vi "Main.vi"() -> ()   [LabVIEW 2018, in "Settings.lvlib"]
doc: "This template is based off of the Queued Message Handler design pattern and the Queued Message Handler project template that ships with LabVIEW.\n\nThe main difference is that the queue is private to this module and communication between modules is performed via Broadcast and Request events.\n\nRequest events are wrapped in public API methods and are handled in the Event Handling Loop (EHL) of this VI. Any module can register for Broadcast events sent by this module. The EHL generates messages based on user interface actions.\n\nThe Message Handling Loop (MHL) processes messages generated by the EHL, or by other messages. The messages are string values, so new messages can be added easily to the Message Cases case structure in the MHL. Each message cluster can also provide an optional value for Message Data, which is a variant that can be converted to whatever message-specific data is required.\n_____\nBased on Delacor QMH Project Template 4.2.1.64."
uses:
  Settings.lvlib
  <vilib>/Delacor/Delacor QMH/Libraries/Module Admin_class/Delacor_lib_QMH_Module Admin.lvclass
  Private API/Data.lvclass
  <vilib>/Delacor/Delacor QMH/Libraries/Message Queue_class/Delacor_lib_QMH_Message Queue.lvclass/Delacor_lib_QMH_Message Queue.ctl
  Stop Argument--cluster.ctl
  <vilib>/Delacor/Delacor QMH/Libraries/Module Admin_class/Delacor_lib_QMH_Module Admin.lvclass/Delacor_lib_QMH_Module Admin.ctl
  Load Settings from File Argument--cluster.ctl
  Instant Load Settings from File Argument--cluster.ctl
  Instant Load Settings from File (Reply Payload)--cluster.ctl
  Common/Typedefs/CTL_Settings_cluster_2.ctl
  SubVi's/Controls/CTL_Histogram_parameters.ctl
  SubVi's/Controls/CTL_Filter_selector.ctl
  SubVi's/Controls/CTL_Acquisition_speed_selector.ctl
  Common/Typedefs/CTL_Segmented_plot_parameters_2.ctl
  Cage Diagram/Typedefs/CTL_Cage_type.ctl
  SubVi's/Controls/CTL_Cage_all_segmentation_params_set.ctl
  SubVi's/Controls/CTL_IO_params_cluster.ctl
  SubVi's/Controls/CTL_Conditions_Array.ctl
  SubVi's/Controls/CTL_Conditions_Cluster.ctl
  SubVi's/Controls/CTL_Condition_type.ctl
  SubVi's/Controls/CTL_Comparison_type.ctl
  SubVi's/Controls/CTL_Validity_check_criteria.ctl
  SubVi's/Controls/CTL_Response_info.ctl
  SubVi's/Controls/CTL_Condition_response_type.ctl
  SubVi's/Controls/CTL_Reponse_port_info.ctl
  SubVi's/Controls/CTL_Calibration_parameters.ctl
  SubVi's/Controls/CTL_Dispenser_calibration_info.ctl
  <vilib>/Utility/miscctls.llb/LVPointTypeDef.ctl
  Private API/Data.lvclass/Data.ctl
  <vilib>/Delacor/Delacor QMH/Libraries/Message Queue_class/Delacor_lib_QMH_Enqueue Message (Single).vi
  <vilib>/Delacor/Delacor QMH/Libraries/Module Admin_class/Delacor_lib_QMH_Get External Launch.vi
  Private API/Methods/Write Status.vi
  <vilib>/Utility/error.llb/Error Cluster From Error Code.vi
  <vilib>/ErrorRing/Error Ring.xnode
  <vilib>/Delacor/Delacor QMH/Libraries/Message Queue_class/Delacor_lib_QMH_Message Queue.lvclass
  Common_Resources.lvlib
  Cage Diagram/Cage Diagram.lvlib
panel:
  out "Settings path to load":path
  in  "Simulate MHL Error":bool
  in  "Simulate EHL Error":bool
  out "error out":errorcluster
  in  "Module Admin":refnum<class "Delacor_lib_QMH_Module Admin.lvclass">
  out "Status":string
  # "Settings Module"
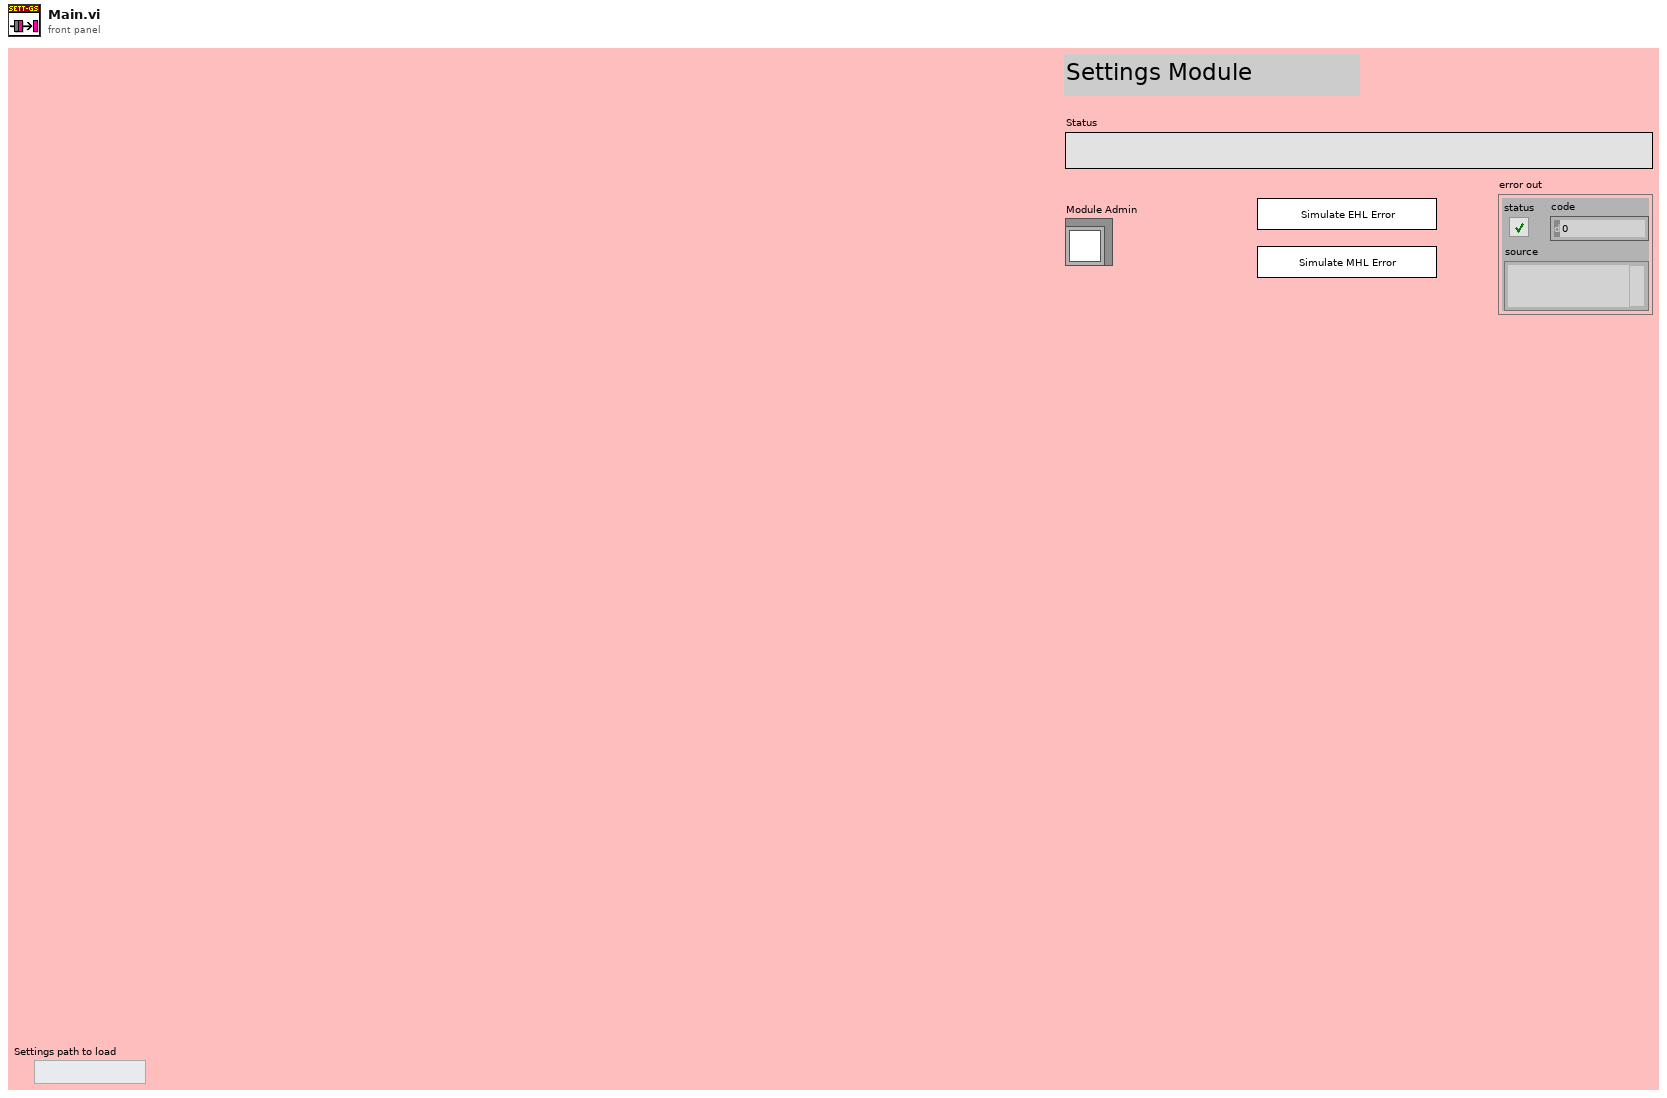
[diagram p1: front panel]
types:
  T1 = typedef "Settings.lvlib/Request Events--cluster.ctl" = cluster{"Stop Module":refnum<user-event>, "Show Panel":refnum<user-event>, "Hide Panel":refnum<user-event>, "Get Module Execution Status":refnum<user-event>, "Show Diagram":refnum<user-event>, "Load Settings from File":refnum<user-event>, "Instant Load Settings from File":refnum<user-event>}
  T2 = enum32{"invalid lock state", "Not Locked", "Locked (No Password)", "Password-protected"}
  T3 = typedef "Settings.lvlib/Stop Argument--cluster.ctl" = cluster{"Origin":string, "Exit via Stop Module Req?":bool, "Wait for Module to stop?":bool}
  T4 = typedef "Settings.lvlib/Load Settings from File Argument--cluster.ctl" = cluster{"Path: Default or Custom?":bool, "Settings File Path":path, "Researcher name":string}
  T5 = typedef "Settings.lvlib/Instant Load Settings from File Argument--cluster.ctl" = cluster{"Path: Default or Custom?":bool, "Settings File Path":path, "Researcher name":string, "Wait Notifier":refnum<notifier>, "wait for reply":bool}
  T6 = typedef "LVPointTypeDef.ctl" = cluster{"Horizontal":i16, "Vertical":i16}
  T7 = enum32{"Invalid", "Standard", "Closed", "Hidden", "Minimized", "Maximized"}
  T8 = typedef "Settings.lvlib/Instant Load Settings from File (Reply Payload)--cluster.ctl" = cluster{"Settings cluster":T9, "Instant Load Settings from File_error":errorcluster}
  T9 = typedef "Common_Resources.lvlib/CTL_Settings_cluster_2.ctl" = cluster{"Defaults":cluster{"Default User":dbl, "VISA Resource Name ":string, "Histogram parameters":T10}, "Recording and saving":cluster{"Researcher name":string, "Name prefix":string, "Data post-processing":T11, "Stop at":dbl, "\"Stop at\" enabled":bool, "Default save folder path":path, "Acquisition FPS":T12}, "Geometry":T13, "IO parameters":T16, "Conditions presets array":T17, "Calibration parameters":T25}
  T10 = typedef "Common_Resources.lvlib/CTL_Histogram_parameters.ctl" = cluster{"max":dbl, "min":dbl, "# bins":i32, "threshold":dbl, "thr. type":enum16{"higher accepted", "lower accepted"}}
  T11 = typedef "Common_Resources.lvlib/CTL_Filter_selector.ctl" = cluster{"Filter type":enum16{"None", "Savitzky-Golay"}, "Length":i32, "Order":i32}
  T12 = typedef "Common_Resources.lvlib/CTL_Acquisition_speed_selector.ctl" = enum16{"Max", "Optimal", "Eco"}
  T13 = typedef "Common_Resources.lvlib/CTL_Segmented_plot_parameters_2.ctl" = cluster{"Sensor board size":enum16{"", "Large"}, "Bridge swap":bool, "Twisted neck":bool, "Bridge H. offset":sgl, "Bridge V. offset":sgl, "Magnets orientation":sgl, "Cage type":T14, "Cage parameters":T15}
  T14 = typedef "Cage Diagram.lvlib/CTL_Cage_type.ctl" = u16
  T15 = typedef "Common_Resources.lvlib/CTL_Cage_all_segmentation_params_set.ctl" = cluster{"Round":variant, "Square":variant, "Donut-maze":variant, "T-maze":variant, "Sociability-maze":variant}
  T16 = typedef "Common_Resources.lvlib/CTL_IO_params_cluster.ctl" = cluster{"IO general config.":u16, "IO 1 configuration":u16, "IO 2 configuration":u16, "IO 3 configuration":u16, "IO 4 configuration":u16, "Activate ext. RS-232":u16, "IO inversion config.":u16, "Sync capability":u8}
  T17 = typedef "Common_Resources.lvlib/CTL_Conditions_Array.ctl" = T18[]
  T18 = typedef "Common_Resources.lvlib/CTL_Conditions_Cluster.ctl" = cluster{"Enabled":bool, "Name":string, "Specifier(s)":cluster{"Specifier enabled":bool, "Condition type":T19, "Comparison type":T20, "Value":dbl, "Validity criteria(s)":cluster{"V. check enabled":bool, "Criteria":T21, "Validity value":dbl}[]}[], "Response":T22, "Has been set":bool}
  T19 = typedef "Common_Resources.lvlib/CTL_Condition_type.ctl" = enum16{"Speed", "Zone", "Angle to wall"}
  T20 = typedef "Common_Resources.lvlib/CTL_Comparison_type.ctl" = enum16{"Less", "Less or Equal", "Equal", "Greater or Equal", "Greater", "Not Equal"}
  T21 = typedef "Common_Resources.lvlib/CTL_Validity_check_criteria.ctl" = enum16{"Running bout (seconds)", "Running bout (meters)"}
  T22 = typedef "Common_Resources.lvlib/CTL_Response_info.ctl" = cluster{"Response type":T23, "TTL port":T24, "TTL pulse length, ms":dbl}
  T23 = typedef "Common_Resources.lvlib/CTL_Condition_response_type.ctl" = enum16{"None", "Air puff", "Liquid reward", "TTL pulse", "TTL pulse (ubr)", "TTL signal"}
  T24 = typedef "Common_Resources.lvlib/CTL_Reponse_port_info.ctl" = enum16{"Port 1", "Port 2", "Port 3", "Port 4"}
  T25 = typedef "Common_Resources.lvlib/CTL_Calibration_parameters.ctl" = cluster{"Timing calibration sw/hw":dbl, "True FPS":dbl, "True frame time, s":dbl, "Disp. calibration info":T26}
  T26 = typedef "Common_Resources.lvlib/CTL_Dispenser_calibration_info.ctl" = cluster{"Channel":u8, "Speed, µl per ms":dbl}[]
  T27 = enum32{"invalid app kind", "Development System", "Run Time System", "Student Edition", "Embedded LabVIEW", "Evaluation", "Custom"}
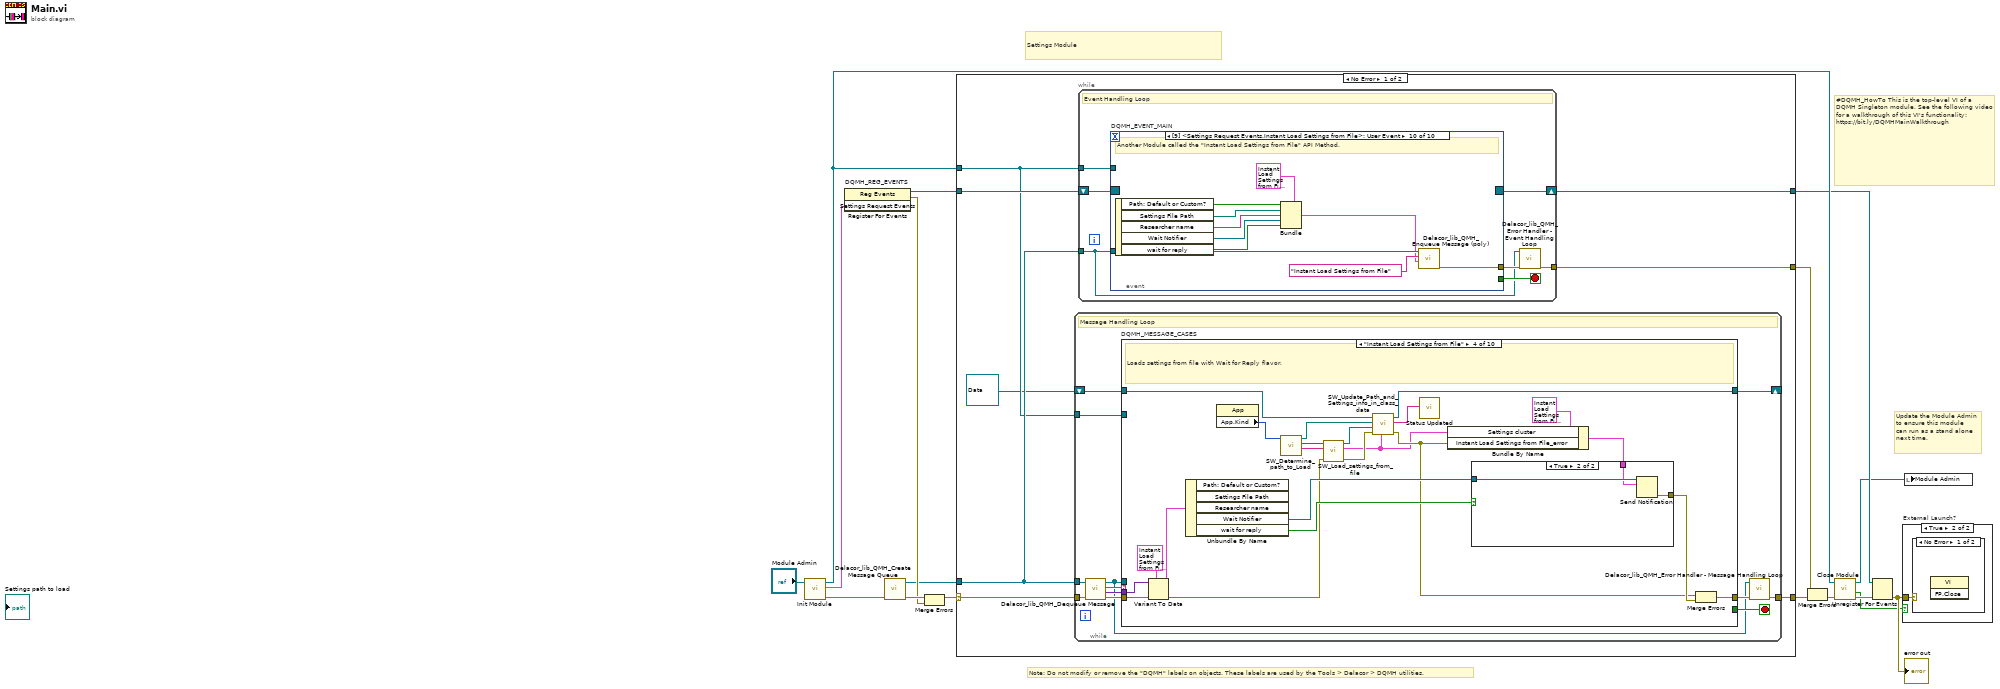
[diagram p0: block diagram]
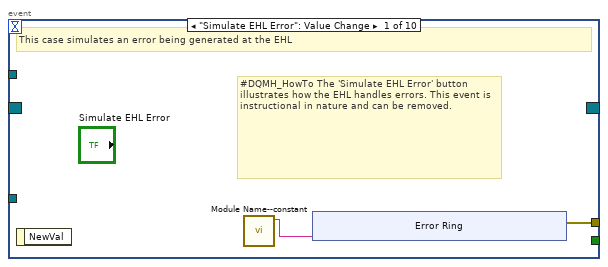
[diagram p2: hidden frame]
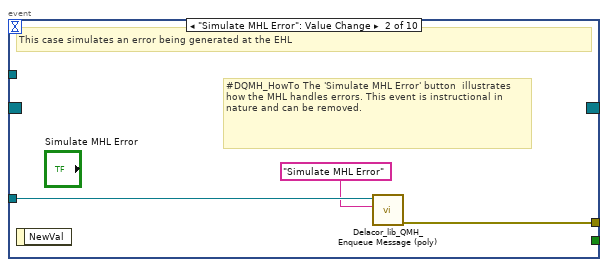
[diagram p3: hidden frame]
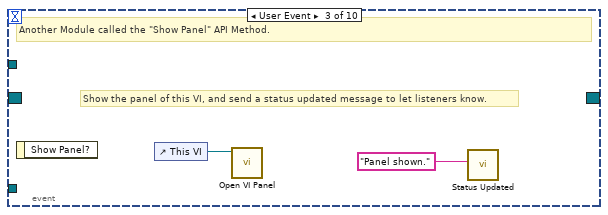
[diagram p4: hidden frame]
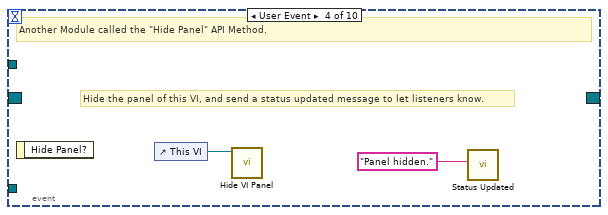
[diagram p5: hidden frame]
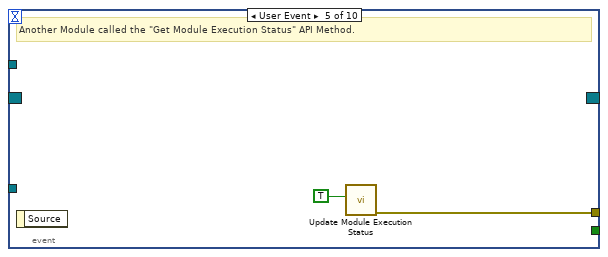
[diagram p6: hidden frame]
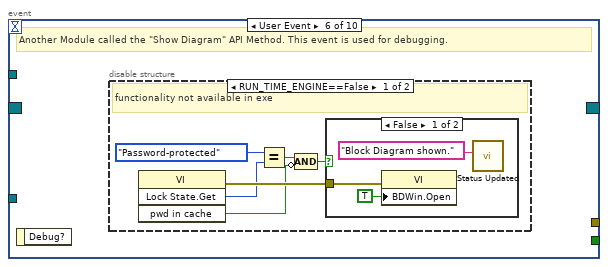
[diagram p7: hidden frame]
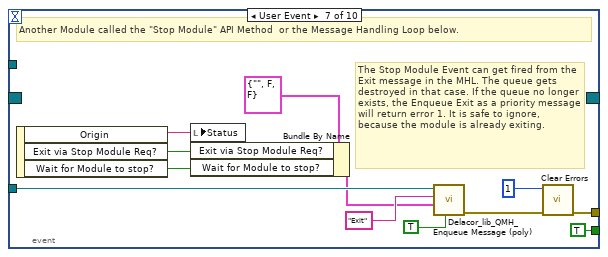
[diagram p10: hidden frame]
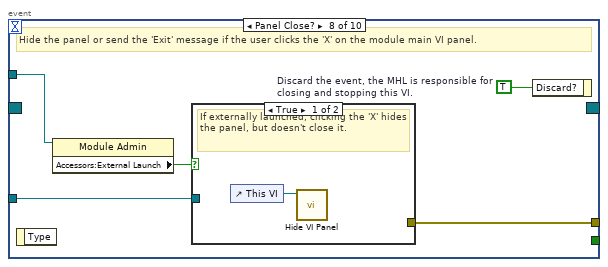
[diagram p11: hidden frame]
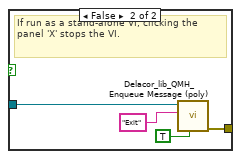
[diagram p12: hidden frame]
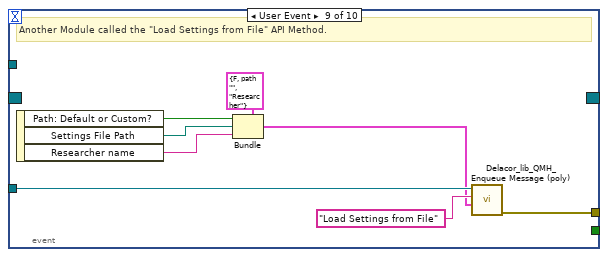
[diagram p13: hidden frame]
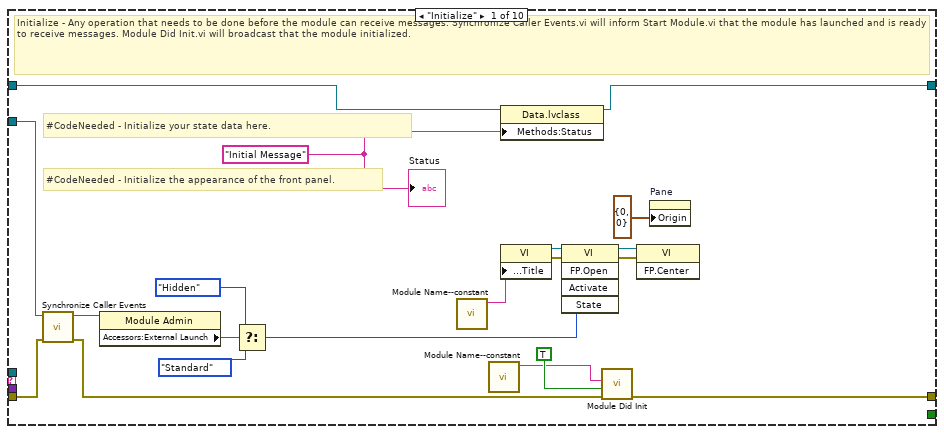
[diagram p14: hidden frame]
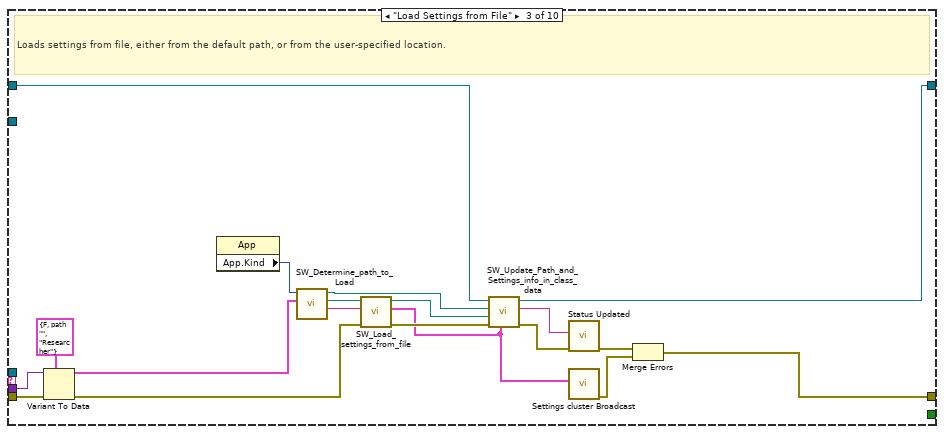
[diagram p16: hidden frame]
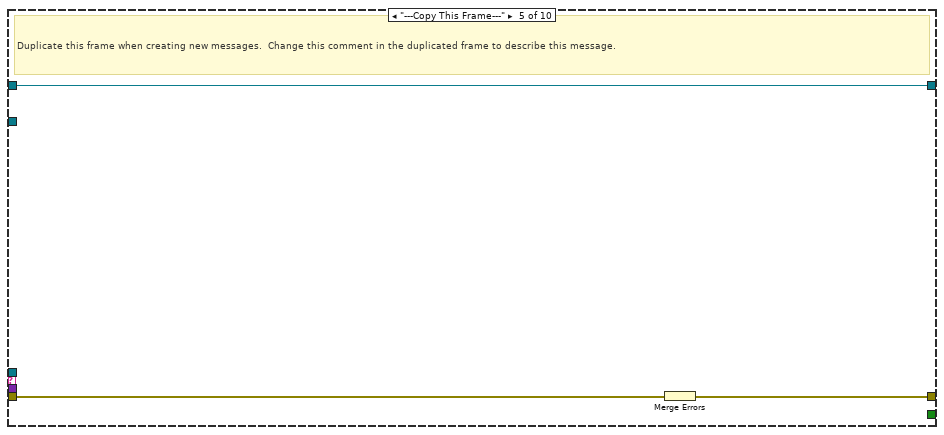
[diagram p18: hidden frame]
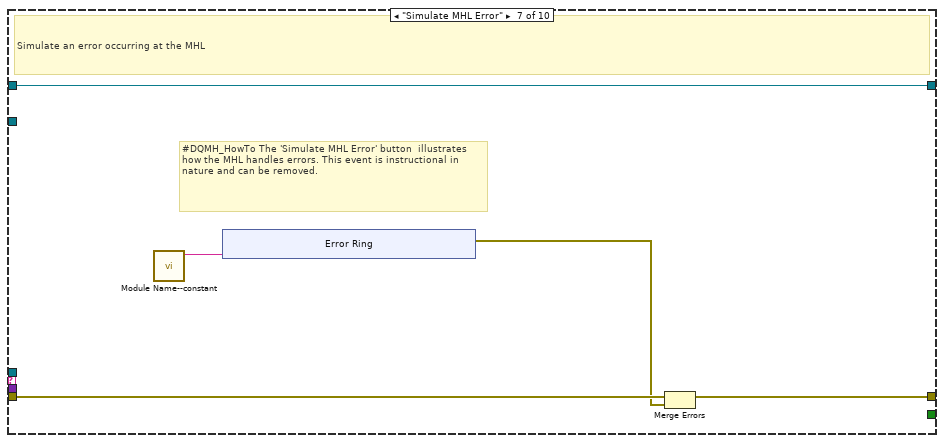
[diagram p20: hidden frame]
diagram:
  # "Settings Module"
  # "#DQMH_HowTo This is the top-level VI of a DQMH Singleton module. See the following video for a walkthrough of this VI's functionality: https://bit.ly/DQMHMainWalkthrough"
  # "Note: Do not modify or remove the \"DQMH\" labels on objects. These labels are used by the Tools > Delacor > DQMH utilities."
  # "Update the Module Admin to ensure this module can run as a stand alone next time."
  n1 = call "Init Module.vi"("Singleton Module Admin in"="Module Admin") -> ("error out"=w16:errorcluster, "Settings Request Events"=w5:T1, "Singleton Module Admin out"=w8:refnum<class "Delacor_lib_QMH_Module Admin.lvclass">)  [unwired: 8 in]
  n2 = register-events "DQMH_REG_EVENTS"(w5) -> (reference out=w6:refnum<event-registration>, error out=w9:errorcluster)  [unwired: 2 in]
  n3 = call <vilib>:"Delacor_lib_QMH_Create Message Queue.vi"("error in (no error)"=w16) -> ("error out"=w11:errorcluster, "Message Queue"=w4:refnum<class "Delacor_lib_QMH_Message Queue.lvclass">)  [unwired: 9 in]
  n4 = Merge Errors(w11, w9) -> (w10:errorcluster)
  n5 = case shown="No Error" w10 {
    selector: w10 -> [w23 w247]
    tunnel: [w25 w247] -> w17
    tunnel: [w22 w244] -> w7
    tunnel: w6 -> [w21 w244]
    tunnel: w4 -> [w20 _]
    tunnel: [w24 _] -> w14
    tunnel: w8 -> [w19 w240]
    frame No Error {
      n6 = while {
        tunnel: w20 -> [w102]
        shift-right: [w106] -> _
        shift-left: refnum<class "Data.lvclass"> refnum ("Settings.lvlib:Data.lvclass") -> [w107]
        tunnel: w23 -> [w110]
        tunnel: [w108] -> w25
        tunnel: w19 -> [w100]
        stop <- w105 stop-if-true
        # "Message Handling Loop"
        n7 = call-dynamic "Delacor_lib_QMH_Dequeue Message.vi"("error in (no error)"=w110, "Message Queue in"=w102) -> ("error out"=w109:errorcluster, "Message Data"=w103:variant, "Message"=w104:string, "Message Queue out"=w101:refnum<class "Delacor_lib_QMH_Message Queue.lvclass">)  [unwired: 6 in]
        n8 = case "DQMH_MESSAGE_CASES" shown="\"Instant Load Settings from File\"" w104 {
          selector: w104 -> [_ _ _ _ _ _ _ _ _ w227]
          tunnel: w101 -> [_ _ _ _ _ _ _ w197 w219 _]
          tunnel: w109 -> [w129 w133 w152 w174 w180 w182 w187 w204 w225 w229]
          tunnel: [w127 w133 w135 w168 w179 w182 w186 w200 w222 w230] -> w111
          tunnel: w107 -> [w114 w132 w143 w158 w178 w181 w184 w199 w218 w228]
          tunnel: [w113 w132 w142 w157 w178 w181 w184 w199 w218 w228] -> w106
          tunnel: [_ _ _ _ _ _ _ _ w217 _] -> w105
          tunnel: w103 -> [_ _ w151 w173 _ _ _ w198 w216 _]
          tunnel: w100 -> [w119 _ _ _ _ _ _ w196 w211 _]
          frame "Initialize" {
            w112 = "Initial Message" ("Initial Message")
            # "#CodeNeeded - Initialize the appearance of the front panel."
            # "#CodeNeeded - Initialize your state data here."
            # "Initialize - Any operation that needs to be done before the module can receive messages. Synchronize Caller Events.vi will inform Start Module.vi that the module has launched and is ready to receive messages. Module Did Init.vi will broadcast that the module initialized."
            n9 = call "Synchronize Caller Events.vi"("error in (no error)"=w129, "Singleton Module Admin in"=w119) -> ("error out"=w128:errorcluster, "Singleton Module Admin out"=w116:refnum<class "Delacor_lib_QMH_Module Admin.lvclass">)  [unwired: 8 in]
            n10 = property class="Module Admin"(reference=w116) -> ("Accessors:External Launch"=w123:bool)  [unwired: 1 in, 2 out]
            n11 = Select(t=T7."Hidden" ("State"), s=w123, f=T7."Standard" ("State")) -> (s? t:f=w120:T7)
            n12 = call "Module Name--constant.vi"() -> ("Module Name"=w126:string)  [unwired: 11 in]
            n13 = call "Module Name--constant.vi"() -> ("Module Name"=w117:string)  [unwired: 11 in]
            n14 = property class="Data.lvclass"(reference=w114, "Methods:Status"=w112) -> (reference out=w113:refnum<class "Data.lvclass">)  [unwired: 1 in, 1 out]
            n15 = property class="VI"("Front Panel.Title"=w126) -> (reference out=w125:refnum<vi>, error out=w131:errorcluster)  [unwired: 2 in]
            n16 = invoke class="VI" method="FP.Open"(reference=w125, error in=w131, "State"=w120) -> (reference out=w124:refnum<vi>, error out=w130:errorcluster)  [unwired: 2 in, 3 out]
            n17 = call "Module Did Init.vi"("error in (no error)"=w128, "Initialized?"=TRUE, "Origin"=w117) -> ("error out"=w127:errorcluster)  [unwired: 8 in]
            n18 = invoke class="VI" method="FP.Center"(reference=w124, error in=w130) -> ()  [unwired: 1 in, 3 out]
            n19 = property on="Pane" class="Pane"("Origin"=T6 {"Horizontal"=0, "Vertical"=0}) -> ()  [unwired: 2 in, 2 out]
            "Status" <- w112
          }
          frame "--- Module Specific ---" {
            # "Separator -- The following cases handle messages specific to this Module."
          }
          frame "Load Settings from File" {
            # "Loads settings from file, either from the default path, or from the user-specified location."
            n20 = Variant To Data(error in=w152, type=T4 {"Path: Default or Custom?"=FALSE, "Settings File Path"=path "", "Researcher name"="Researcher"} ("Load Settings from File Argument"), Variant=w151) -> (data=w149:T4, error out=w147:errorcluster)
            n21 = property class="App"() -> ("App.Kind"=w148:T27)  [unwired: 2 in, 2 out]
            n22 = call "SW_Determine_path_to_Load.vi"("Load Settings from File Argument"=w149, "App.Kind"=w148) -> ("Researcher name"=w145:string, "User Settings path"=w146:path, "Program Settings path"=w138:path)  [unwired: 7 in]
            n23 = call "SW_Load_settings_from_file.vi"("error in (no error)"=w147, "Researcher name in"=w145, "Settings path in"=w146) -> ("Error Out"=w144:errorcluster, "Settings cluster out"=w136:T9, "Settings file path out"=w137:path)  [unwired: 4 in]
            n24 = call "SW_Update_Path_and_Settings_info_in_class_data.vi"("Settings cluster in"=w136, "error in (no error)"=w144, "Settings file path in"=w137, "Program Settings path"=w138, "Data in"=w143) -> ("error out"=w141:errorcluster, "Status out"=w140:string, "Data out"=w142:refnum<class "Data.lvclass">)  [unwired: 4 in]
            n25 = call "Status Updated.vi"("error in (no error)"=w141, "Status"=w140) -> ("error out"=w139:errorcluster)  [unwired: 9 in]
            n26 = call "Settings cluster Broadcast.vi"("Settings cluster"=w136) -> ("error out"=w134:errorcluster)  [unwired: 10 in]
            n27 = Merge Errors(w139, w134) -> (w135:errorcluster)
          }
          frame "Instant Load Settings from File" {
            # "Loads settings from file with Wait for Reply flavor."
            n28 = Variant To Data(error in=w174, type=T5 {"Path: Default or Custom?"=FALSE, "Settings File Path"=path "", "Researcher name"="Researcher", "Wait Notifier"=refnum, "wait for reply"=FALSE} ("Instant Load Settings from File Argument"), Variant=w173) -> (data=w171:T5, error out=w161:errorcluster)
            n29 = Unbundle By Name(w171) -> ("Wait Notifier"=w165:refnum<notifier>, "wait for reply"=w164:bool)  [unwired: 3 out]
            n30 = property class="App"() -> ("App.Kind"=w166:T27)  [unwired: 2 in, 2 out]
            n31 = call "SW_Determine_path_to_Load.vi"("App.Kind"=w166) -> ("Researcher name"=w162:string, "User Settings path"=w163:path, "Program Settings path"=w155:path)  [unwired: 8 in]
            n32 = call "SW_Load_settings_from_file.vi"("error in (no error)"=w161, "Researcher name in"=w162, "Settings path in"=w163) -> ("Error Out"=w160:errorcluster, "Settings cluster out"=w156:T9, "Settings file path out"=w154:path)  [unwired: 4 in]
            n33 = call "SW_Update_Path_and_Settings_info_in_class_data.vi"("Settings cluster in"=w156, "error in (no error)"=w160, "Settings file path in"=w154, "Program Settings path"=w155, "Data in"=w158) -> ("error out"=w159:errorcluster, "Status out"=w153:string, "Data out"=w157:refnum<class "Data.lvclass">)  [unwired: 4 in]
            n34 = call "Status Updated.vi"("Status"=w153) -> ()  [unwired: 10 in, 1 out]
            n35 = Bundle By Name(cluster=T8 {"Settings cluster"={"Defaults"={"Default User"=0.0, "VISA Resource Name "="Tracker", "Histogram parameters"={"max"=300.0, "min"=0.0, "# bins"=10, "threshold"=8.0, "thr. type"=enum."higher accepted"}}, "Recording and saving"={"Researcher name"="Researcher", "Name prefix"="Track", "Data post-processing"={"Filter type"=enum."Savitzky-Golay", "Length"=31, "Order"=3}, "Stop at"=0.0, "\"Stop at\" enabled"=FALSE, "Default save folder path"=path "", "Acquisition FPS"=enum."Max"}, "Geometry"={"Sensor board size"=enum."Large", "Bridge swap"=FALSE, "Twisted neck"=FALSE, "Bridge H. offset"=30.0, "Bridge V. offset"=75.0, "Magnets orientation"=0.0, "Cage type"=0, "Cage parameters"={"Round"=variant, "Square"=variant, "Donut-maze"=variant, "T-maze"=variant, "Sociability-maze"=variant}}, "IO parameters"={"IO general config."=12, "IO 1 configuration"=1, "IO 2 configuration"=1, "IO 3 configuration"=0, "IO 4 configuration"=0, "Activate ext. RS-232"=0, "IO inversion config."=0, "Sync capability"=1}, "Conditions presets array"=[{"Enabled"=FALSE, "Name"="", "Specifier(s)"=[], "Response"={"Response type"=enum."Air puff", "TTL port"=enum."Port 1", "TTL pulse length, ms"=0.0}, "Has been set"=FALSE}, {"Enabled"=FALSE, "Name"="", "Specifier(s)"=[], "Response"={"Response type"=enum."Air puff", "TTL port"=enum."Port 1", "TTL pulse length, ms"=0.0}, "Has been set"=FALSE}, {"Enabled"=FALSE, "Name"="", "Specifier(s)"=[], "Response"={"Response type"=enum."Air puff", "TTL port"=enum."Port 1", "TTL pulse length, ms"=0.0}, "Has been set"=FALSE}, {"Enabled"=FALSE, "Name"="", "Specifier(s)"=[], "Response"={"Response type"=enum."Air puff", "TTL port"=enum."Port 1", "TTL pulse length, ms"=0.0}, "Has been set"=FALSE}, {"Enabled"=FALSE, "Name"="", "Specifier(s)"=[], "Response"={"Response type"=enum."Air puff", "TTL port"=enum."Port 1", "TTL pulse length, ms"=0.0}, "Has been set"=FALSE}, {"Enabled"=FALSE, "Name"="", "Specifier(s)"=[], "Response"={"Response type"=enum."Air puff", "TTL port"=enum."Port 1", "TTL pulse length, ms"=0.0}, "Has been set"=FALSE}, {"Enabled"=FALSE, "Name"="", "Specifier(s)"=[], "Response"={"Response type"=enum."Air puff", "TTL port"=enum."Port 1", "TTL pulse length, ms"=0.0}, "Has been set"=FALSE}, {"Enabled"=FALSE, "Name"="", "Specifier(s)"=[], "Response"={"Response type"=enum."Air puff", "TTL port"=enum."Port 1", "TTL pulse length, ms"=0.0}, "Has been set"=FALSE}, {"Enabled"=FALSE, "Name"="", "Specifier(s)"=[], "Response"={"Response type"=enum."Air puff", "TTL port"=enum."Port 1", "TTL pulse length, ms"=0.0}, "Has been set"=FALSE}, {"Enabled"=FALSE, "Name"="", "Specifier(s)"=[], "Response"={"Response type"=enum."Air puff", "TTL port"=enum."Port 1", "TTL pulse length, ms"=0.0}, "Has been set"=FALSE}, {"Enabled"=FALSE, "Name"="", "Specifier(s)"=[], "Response"={"Response type"=enum."Air puff", "TTL port"=enum."Port 1", "TTL pulse length, ms"=0.0}, "Has been set"=FALSE}, {"Enabled"=FALSE, "Name"="", "Specifier(s)"=[], "Response"={"Response type"=enum."Air puff", "TTL port"=enum."Port 1", "TTL pulse length, ms"=0.0}, "Has been set"=FALSE}, {"Enabled"=FALSE, "Name"="", "Specifier(s)"=[], "Response"={"Response type"=enum."Air puff", "TTL port"=enum."Port 1", "TTL pulse length, ms"=0.0}, "Has been set"=FALSE}, {"Enabled"=FALSE, "Name"="", "Specifier(s)"=[], "Response"={"Response type"=enum."Air puff", "TTL port"=enum."Port 1", "TTL pulse length, ms"=0.0}, "Has been set"=FALSE}], "Calibration parameters"={"Timing calibration sw/hw"=1.0, "True FPS"=80.0, "True frame time, s"=0.0125, "Disp. calibration info"=[]}}, "Instant Load Settings from File_error"={"status"=FALSE, "code"=0, "source"=""}} ("Instant Load Settings from File (Reply Payload)"), "Settings cluster"=w156, "Instant Load Settings from File_error"=w159) -> (w170:T8)
            n36 = case shown="True" w164 {
              tunnel: w165 -> [_ w177]
              tunnel: w170 -> [_ w176]
              tunnel: [_ w175] -> w167
              frame False {
              }
              frame True {
                n37 = Send Notification(notification=w176, notifier=w177) -> (error out=w175:errorcluster)  [unwired: 1 in, 1 out]
              }
            }
            n38 = Merge Errors(w159, w167) -> (w168:errorcluster)
          }
          frame "---Copy This Frame---" {
            # "Duplicate this frame when creating new messages.  Change this comment in the duplicated frame to describe this message."
            n39 = Merge Errors(w180) -> (w179:errorcluster)
          }
          frame "--- Exit and Error Handling---" {
            # "Separator - The following cases handle errors and exit messages."
          }
          frame "Simulate MHL Error" {
            # "#DQMH_HowTo The 'Simulate MHL Error' button  illustrates how the MHL handles errors. This event is instructional in nature and can be removed."
            # "Simulate an error occurring at the MHL"
            n40 = call "Module Name--constant.vi"() -> ("Module Name"=w183:string)  [unwired: 11 in]
            n41 = xnode "Error Ring"("parameter 0"=w183) -> ("error out"=w185:errorcluster)
            n42 = Merge Errors(w187, w185) -> (w186:errorcluster)
          }
          frame "Error" {
            # "#CodeRecommended - If you ever change the name of this \"Error\" message, you'll need to update the name in the Check Loop Error.vi as well."
            # "#CodeRecommended - If the module is running in standalone mode (External Launch = FALSE), this code will pop up an error dialog and call the 'Exit' message if an error occurs. Add more fine-grained error handling here."
            # "Error - Check the error message data and respond accordingly. This message is sent by the \"Error Handler\" VIs at the end of each loop in this application."
            n43 = property class="Module Admin"(reference=w196) -> ("Accessors:External Launch"=w195:bool)  [unwired: 1 in, 2 out]
            n44 = Variant To Data(error in=w204, type=errorcluster {"status"=FALSE, "code"=0, "source"=""} ("error constant"), Variant=w198) -> (data=w205:errorcluster, error out=w202:errorcluster)
            n45 = call "Error Reported.vi"("Error"=w205) -> ()  [unwired: 10 in, 1 out]
            n46 = case shown="False" w195 {
              tunnel: [w210 _] -> w201
              tunnel: w197 -> [w208 _]
              tunnel: w205 -> [w209 _]
              frame False {
                # "If the module is running standalone, then pop up an error dialog and call the \"Exit\" message."
                n47 = call <vilib>:"Simple Error Handler.vi"("error in (no error)"=w209) -> ()  [unwired: 4 in, 5 out]
                n48 = call-poly <vilib>:"Delacor_lib_QMH_Enqueue Message (poly).vi"("Priority Message? (F)"=TRUE, "Message"="Exit", "Message Queue in"=w208) -> ("error out"=w210:errorcluster)  [unwired: 7 in, 1 out]
              }
              frame True {
                # "If the module was launched externally, calling the Error Reported broadcast VI is the only action performed by the \"Error\" message. The module's caller can then process the error appropriately."
              }
            }
            n49 = Merge Errors(w202, w201) -> (w200:errorcluster)
            n50 = local write "error out"(w200) -> ()
          }
          frame "Exit" {
            w215 = 91  # 91: not all Exit messages will have an argument
            w217 = TRUE  # Stop the VI
            # "Release the message queue reference"
            # "#CodeNeeded - Add any required cleanup code here"
            # "Exit - Exit the application."
            n51 = Variant To Data(error in=w225, type=T3 {"Origin"="", "Exit via Stop Module Req?"=FALSE, "Wait for Module to stop?"=FALSE} ("Stop Argument"), Variant=w216) -> (data=w213:T3, error out=w221:errorcluster)
            n52 = call <vilib>:"Clear Errors.vi"("error in (no error)"=w221, "specific error code to clear (0: all)"=w215) -> ("error out"=w224:errorcluster)  [unwired: 4 in, 1 out]
            n53 = control-ref of="This VI"() -> (w212:refnum<vi>)
            n54 = call-dynamic "Delacor_lib_QMH_Release Message Queue.vi"("error in (no error)"=w224, "Message Queue"=w219) -> ("error out"=w223:errorcluster)  [unwired: 9 in]
            n55 = call "Handle Exit.vi"("Stop Argument"=w213, "Admin in"=w211, "VI reference"=w212) -> ("error out"=w220:errorcluster)  [unwired: 7 in, 1 out]
            n56 = Merge Errors(w223, w220) -> (w222:errorcluster)
          }
          frame Default {
            # "'Default' case only runs if there is a message that isn't defined in any of the other cases.  Output a programming error."
            n57 = call "Module Name--constant.vi"() -> ("Module Name"=w226:string)  [unwired: 11 in]
            n58 = xnode "Error Ring"("parameter 0"=w227, "parameter 1"=w226) -> ("error out"=w231:errorcluster)
            n59 = Merge Errors(w229, w231) -> (w230:errorcluster)
          }
        }
        n60 = call-dynamic "Delacor_lib_QMH_Error Handler - Message Handling Loop.vi"("error in (no error)"=w111, "Message Queue in"=w101) -> ("dup error in"=w108:errorcluster)  [unwired: 8 in, 1 out]
      }
      n61 = while {
        tunnel: w20 -> [w26]
        shift-right: [w29] -> w22
        shift-left: w21 -> [w30]
        tunnel: [w31] -> w24
        tunnel: w19 -> [w27]
        stop <- w28 stop-if-true
        # "Event Handling Loop"
        n62 = event "DQMH_EVENT_MAIN" shown="[9] <Settings Request Events.Instant Load Settings from File>: User Event" {
          selector: w30 -> [_ _ _ _ _ _ _ _ _ _]
          dyn-events: [_ _ _ _ _ _ _ _ _ _] -> w29
          timeout: _ -> [_ _ _ _ _ _ _ _ _ _]
          tunnel: [_ _ _ _ _ _ TRUE ("Discard?") _ _ _] -> w28
          tunnel: w26 -> [_ w43 _ _ _ _ w67 w74 w89 w99]
          tunnel: [w34 w44 _ _ w50 _ w70 w76 w84 w93] -> w32
          tunnel: w27 -> [_ _ _ _ _ _ _ w73 _ _]
          event "Simulate EHL Error": Value Change {
            # "#DQMH_HowTo The 'Simulate EHL Error' button  illustrates how the EHL handles errors. This event is instructional in nature and can be removed."
            # "This case simulates an error being generated at the EHL"
            n63 = event-data() -> ()  [unwired: 1 in, 1 out]
            n64 = call "Module Name--constant.vi"() -> ("Module Name"=w33:string)  [unwired: 11 in]
            n65 = xnode "Error Ring"("parameter 0"=w33) -> ("error out"=w34:errorcluster)
          }
          event "Simulate MHL Error": Value Change {
            # "#DQMH_HowTo The 'Simulate MHL Error' button  illustrates how the MHL handles errors. This event is instructional in nature and can be removed."
            # "This case simulates an error being generated at the EHL"
            n66 = event-data() -> ()  [unwired: 1 in, 1 out]
            n67 = call-poly <vilib>:"Delacor_lib_QMH_Enqueue Message (poly).vi"("Message"="Simulate MHL Error", "Message Queue in"=w43) -> ("error out"=w44:errorcluster)  [unwired: 8 in, 1 out]
          }
          event User Event {
            # "Show the panel of this VI, and send a status updated message to let listeners know."
            # "Another Module called the \"Show Panel\" API Method."
            n68 = event-data() -> ()  [unwired: 1 in, 1 out]
            n69 = control-ref of="This VI"() -> (w46:refnum<vi>)
            n70 = call "Open VI Panel.vi"("VI"=w46) -> ()  [unwired: 10 in, 1 out]
            n71 = call "Status Updated.vi"("Status"="Panel shown." ("format string")) -> ()  [unwired: 10 in, 1 out]
          }
          event User Event {
            # "Hide the panel of this VI, and send a status updated message to let listeners know."
            # "Another Module called the \"Hide Panel\" API Method."
            n72 = event-data() -> ()  [unwired: 1 in, 1 out]
            n73 = control-ref of="This VI"() -> (w48:refnum<vi>)
            n74 = call "Hide VI Panel.vi"("VI"=w48) -> ()  [unwired: 10 in, 1 out]
            n75 = call "Status Updated.vi"("Status"="Panel hidden." ("format string")) -> ()  [unwired: 10 in, 1 out]
          }
          event User Event {
            # "Another Module called the \"Get Module Execution Status\" API Method."
            n76 = event-data() -> ()  [unwired: 1 in, 1 out]
            n77 = call "Update Module Execution Status.vi"("Running?"=TRUE) -> ("error out"=w50:errorcluster)  [unwired: 10 in]
          }
          event User Event {
            # "Another Module called the \"Show Diagram\" API Method. This event is used for debugging."
            n78 = event-data() -> ()  [unwired: 1 in, 1 out]
            n79 = disable-structure shown="RUN_TIME_ENGINE==False" {
              frame condition #0 (active) {
                # "functionality not available in exe"
                n80 = invoke class="VI" method="Lock State.Get"() -> (error out=w56:errorcluster, "Get Lock State"=w55:T2, "pwd in cache"=w52:bool)  [unwired: 4 in, 1 out]
                n81 = Equal?(x=T2."Password-protected", y=w55) -> (x = y?=w53:bool)
                n82 = Compound Arithmetic op=AND(w53, invert w52) -> (w51:bool)
                n83 = case shown="False" w51 {
                  tunnel: w56 -> [w59 _]
                  frame False {
                    n84 = property class="VI"(error in=w59, "BDWin.Open"=TRUE ("Block Diagram Window:Open")) -> ()  [unwired: 1 in, 2 out]
                    n85 = call "Status Updated.vi"("Status"="Block Diagram shown." ("format string")) -> ()  [unwired: 10 in, 1 out]
                  }
                  frame True {
                    # "Password-protected VI, and the password is not in the cache. Do not show the diagram."
                  }
                }
              }
              frame condition #1 {
              }
            }
          }
          event User Event {
            # "The Stop Module Event can get fired from the Exit message in the MHL. The queue gets destroyed in that case. If the queue no longer exists, the Enqueue Exit as a priority message will return error 1. It is safe to ignore, because the module is already exiting."
            # "Another Module called the \"Stop Module\" API Method  or the Message Handling Loop below."
            n86 = event-data() -> ("Origin"=w66:string, "Exit via Stop Module Req?"=w62:bool, "Wait for Module to stop?"=w61:bool)  [unwired: 1 in]
            n87 = local write "Status"(w66) -> ()
            n88 = Bundle By Name(cluster=T3 {"Origin"="", "Exit via Stop Module Req?"=FALSE, "Wait for Module to stop?"=FALSE} ("Stop Argument"), "Exit via Stop Module Req?"=w62, "Wait for Module to stop?"=w61) -> (w60:T3)
            n89 = call-poly <vilib>:"Delacor_lib_QMH_Enqueue Message (poly).vi"("Priority Message? (F)"=TRUE, "Message Data"=w60, "Message"="Exit", "Message Queue in"=w67) -> ("error out"=w71:errorcluster)  [unwired: 6 in, 1 out]
            n90 = call <vilib>:"Clear Errors.vi"("error in (no error)"=w71, "specific error code to clear (0: all)"=1) -> ("error out"=w70:errorcluster)  [unwired: 4 in, 1 out]
          }
          event Panel Close? {
            w75 = TRUE  # Discard the event, the MHL is responsible for closing and stopping this VI.
            # "Hide the panel or send the 'Exit' message if the user clicks the 'X' on the module main VI panel."
            n91 = event-data() -> ()  [unwired: 1 in, 1 out]
            n92 = property class="Module Admin"(reference=w73) -> ("Accessors:External Launch"=w72:bool)  [unwired: 1 in, 2 out]
            n93 = case shown="True" w72 {
              tunnel: w74 -> [_ w80]
              tunnel: [_ w81] -> w76
              frame True {
                # "If externally launched, clicking the 'X' hides the panel, but doesn't close it."
                n94 = control-ref of="This VI"() -> (w77:refnum<vi>)
                n95 = call "Hide VI Panel.vi"("VI"=w77) -> ()  [unwired: 10 in, 1 out]
              }
              frame False {
                # "If run as a stand-alone VI, clicking the panel 'X' stops the VI."
                n96 = call-poly <vilib>:"Delacor_lib_QMH_Enqueue Message (poly).vi"("Priority Message? (F)"=TRUE, "Message"="Exit", "Message Queue in"=w80) -> ("error out"=w81:errorcluster)  [unwired: 7 in, 1 out]
              }
            }
            n97 = event-data("Discard?"=w75) -> ()  [unwired: 1 in, 1 out]
          }
          event User Event {
            # "Another Module called the \"Load Settings from File\" API Method."
            n98 = event-data() -> ("Path: Default or Custom?"=w85:bool, "Settings File Path"=w83:path, "Researcher name"=w82:string)  [unwired: 1 in]
            n99 = Bundle(cluster=T4 {"Path: Default or Custom?"=FALSE, "Settings File Path"=path "", "Researcher name"="Researcher"} ("Load Settings from File Argument"), "Path: Default or Custom?"=w85, "Settings File Path"=w83, "Researcher name"=w82) -> (w86:T4)
            n100 = call-poly <vilib>:"Delacor_lib_QMH_Enqueue Message (poly).vi"("Message Data"=w86, "Message"="Load Settings from File", "Message Queue in"=w89) -> ("error out"=w84:errorcluster)  [unwired: 7 in, 1 out]
          }
          event User Event {
            # "Another Module called the \"Instant Load Settings from File\" API Method."
            n101 = event-data() -> ("Path: Default or Custom?"=w95:bool, "Settings File Path"=w90:path, "Researcher name"=w91:string, "Wait Notifier"=w92:refnum<notifier>, "wait for reply"=w94:bool)  [unwired: 1 in]
            n102 = Bundle(cluster=T5 {"Path: Default or Custom?"=FALSE, "Settings File Path"=path "", "Researcher name"="Researcher", "Wait Notifier"=refnum, "wait for reply"=FALSE} ("Instant Load Settings from File Argument"), "Path: Default or Custom?"=w95, "Settings File Path"=w90, "Researcher name"=w91, "Wait Notifier"=w92, "wait for reply"=w94) -> (w96:T5)
            n103 = call-poly <vilib>:"Delacor_lib_QMH_Enqueue Message (poly).vi"("Message Data"=w96, "Message"="Instant Load Settings from File", "Message Queue in"=w99) -> ("error out"=w93:errorcluster)  [unwired: 7 in, 1 out]
          }
        }
        n104 = call-dynamic "Delacor_lib_QMH_Error Handler - Event Handling Loop.vi"("error in (no error)"=w32, "Message Queue in"=w26) -> ("dup error in"=w31:errorcluster)  [unwired: 8 in, 1 out]
      }
    }
    frame Error {
      # "Synchronize Caller Events.vi will inform Start Module.vi that the module has launched and will let the code calling Start Module.vi register for broadcasts and would permit the caller receive the broadcast that an error occurred at launch time."
      n105 = call "Synchronize Caller Events.vi"("Singleton Module Admin in"=w240) -> ("error out"=w245:errorcluster)  [unwired: 9 in, 1 out]
      n106 = call "Module Name--constant.vi"() -> ("Module Name"=w243:string)  [unwired: 11 in]
      n107 = Format Into String(format string="An error occurred during initialization. %s is no longer running.", w243) -> (resulting string=w241:string)  [unwired: 2 in, 1 out]
      n108 = Merge Errors(w247, w245) -> (w246:errorcluster)
      n109 = call "Error Reported.vi"("Additional Information"=w241, "Error"=w246) -> ()  [unwired: 9 in, 1 out]
    }
  }
  n110 = Merge Errors(w14, w17) -> (w13:errorcluster)
  n111 = call "Close Module.vi"("error in (no error)"=w13, "Module Admin in"=w8) -> ("error out"=w15:errorcluster, "External Launch"=w1:bool, "Module Admin out"=w2:refnum<class "Delacor_lib_QMH_Module Admin.lvclass">)  [unwired: 7 in]
  n112 = Unregister For Events(event registration refnum=w7, error in=w15) -> (error out=w12:errorcluster)
  "error out" <- w12
  n113 = case "External Launch?" shown="True" w1 {
    tunnel: w12 -> [_ w248]
    frame False {
    }
    frame True {
      n114 = case shown="No Error" w248 {
        frame No Error {
          n115 = invoke class="VI" method="FP.Close"() -> ()  [unwired: 3 in, 3 out]
        }
        frame Error {
          n116 = invoke class="VI" method="FP.Open"("Activate"=TRUE ("Activate?")) -> ()  [unwired: 4 in, 5 out]
        }
      }
    }
  }
  n117 = local write "Module Admin"(w2) -> ()
